vi "move_invader_intensity.vi"(11 "MainCluster_IN":T9) -> (3 "MainCluster_OUT":T9)   [LabVIEW 2019]
uses:
  InitCluster.ctl
  CharacterCluster.ctl
  <vilib>/picture/picture.llb/imagedata.ctl
  ShotInitCluster.ctl
  <vilib>/Utility/miscctls.llb/LVPositionTypeDef.ctl
  <vilib>/Utility/miscctls.llb/LVBoundsTypeDef.ctl
  InvaderPositionArray.ctl
  move_dir_lr.ctl
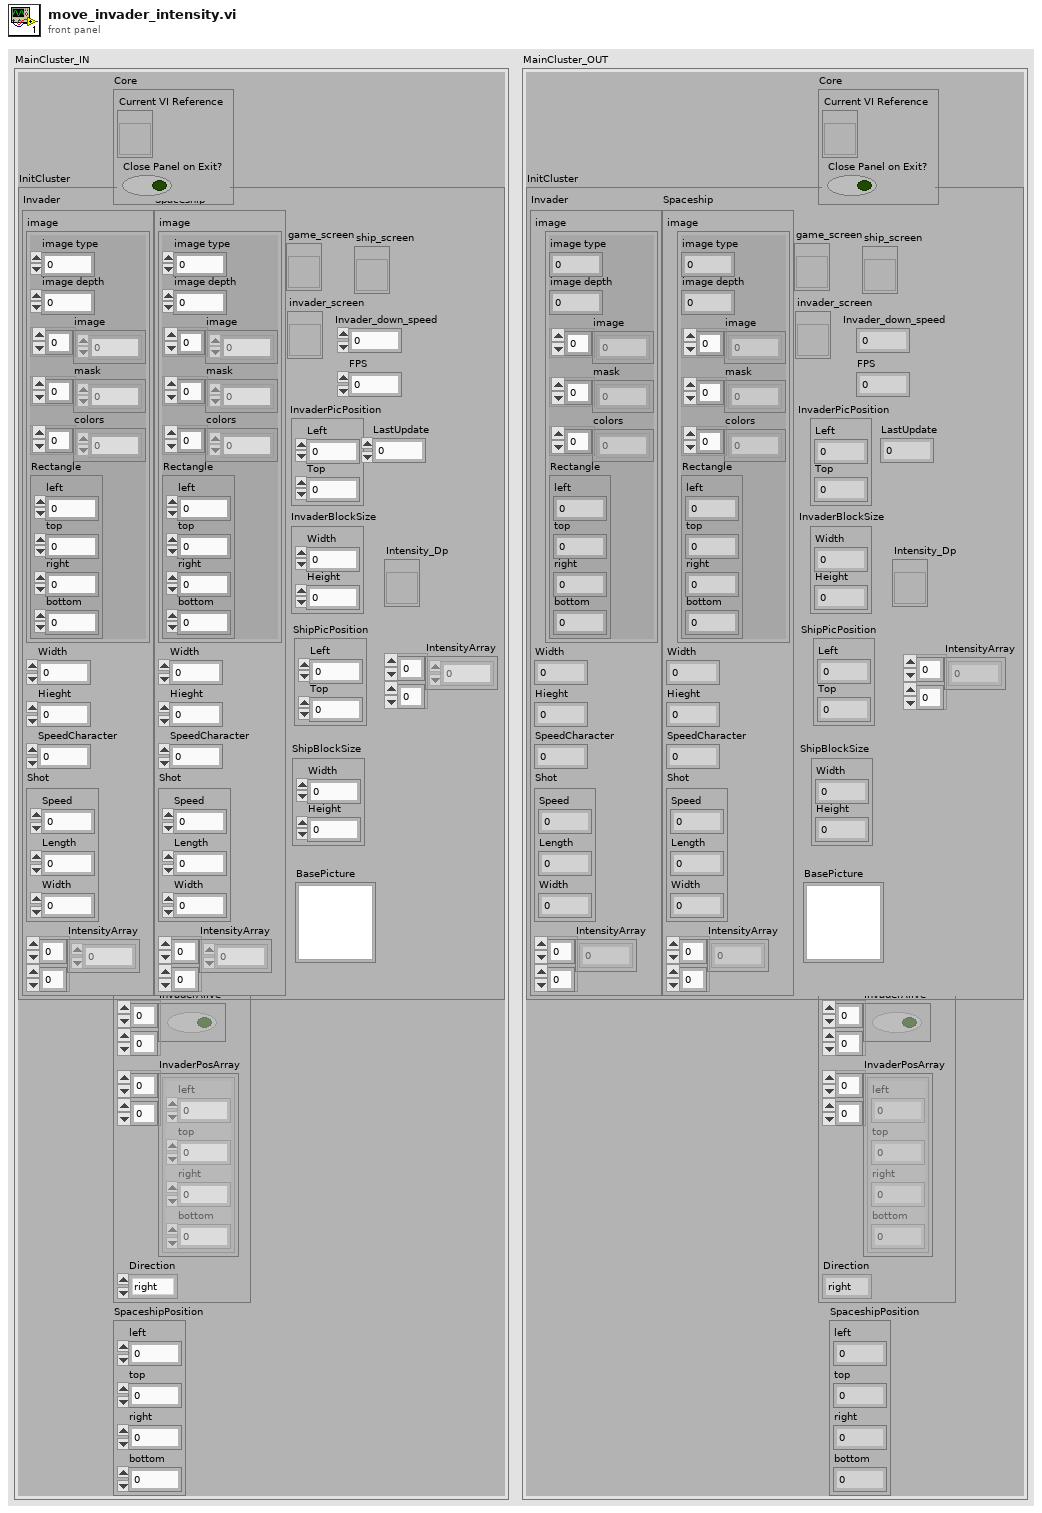
[diagram p1: front panel]
types:
  T1 = typedef "InitCluster.ctl" = cluster{"Invader":T2, "Spaceship":T2, "game_screen":refnum<vi>, "BasePicture":picture, "invader_screen":refnum<vi>, "InvaderPicPosition":T5, "Invader_down_speed":i16, "FPS":u16, "InvaderBlockSize":T6, "ship_screen":refnum<vi>, "ShipBlockSize":T6, "ShipPicPosition":T5, "LastUpdate":u32, "Intensity_Dp":refnum<vi>, "IntensityArray":u8[][]}
  T2 = typedef "CharacterCluster.ctl" = cluster{"image":T3, "Width":u32, "Hieght":u32, "SpeedCharacter":u32, "Shot":T4, "IntensityArray":u8[][]}
  T3 = typedef "imagedata.ctl" = cluster{"image type":i32, "image depth":i32, "image":u8[], "mask":u8[], "colors":u32[], "Rectangle":cluster{"left":i16, "top":i16, "right":i16, "bottom":i16}}
  T4 = typedef "ShotInitCluster.ctl" = cluster{"Speed":u32, "Length":u32, "Width":u32}
  T5 = typedef "LVPositionTypeDef.ctl" = cluster{"Left":i32, "Top":i32}
  T6 = typedef "LVBoundsTypeDef.ctl" = cluster{"Width":u32, "Height":u32}
  T7 = typedef "InvaderPositionArray.ctl" = cluster{"InvaderAlive":bool[][], "InvaderPosArray":cluster{"left":i16, "top":i16, "right":i16, "bottom":i16}[][], "Direction":T8}
  T8 = typedef "move_dir_lr.ctl" = enum16{"right", "left"}
  T9 = cluster{"Core":cluster{"Current VI Reference":refnum<vi>, "Close Panel on Exit?":bool}, "InitCluster":T1, "InvaderPosArray":T7, "SpaceshipPosition":cluster{"left":i16, "top":i16, "right":i16, "bottom":i16}}
  T10 = cluster{"left":i16, "top":i16, "right":i16, "bottom":i16}[][]
  T11 = cluster{"left":i16, "top":i16, "right":i16, "bottom":i16}
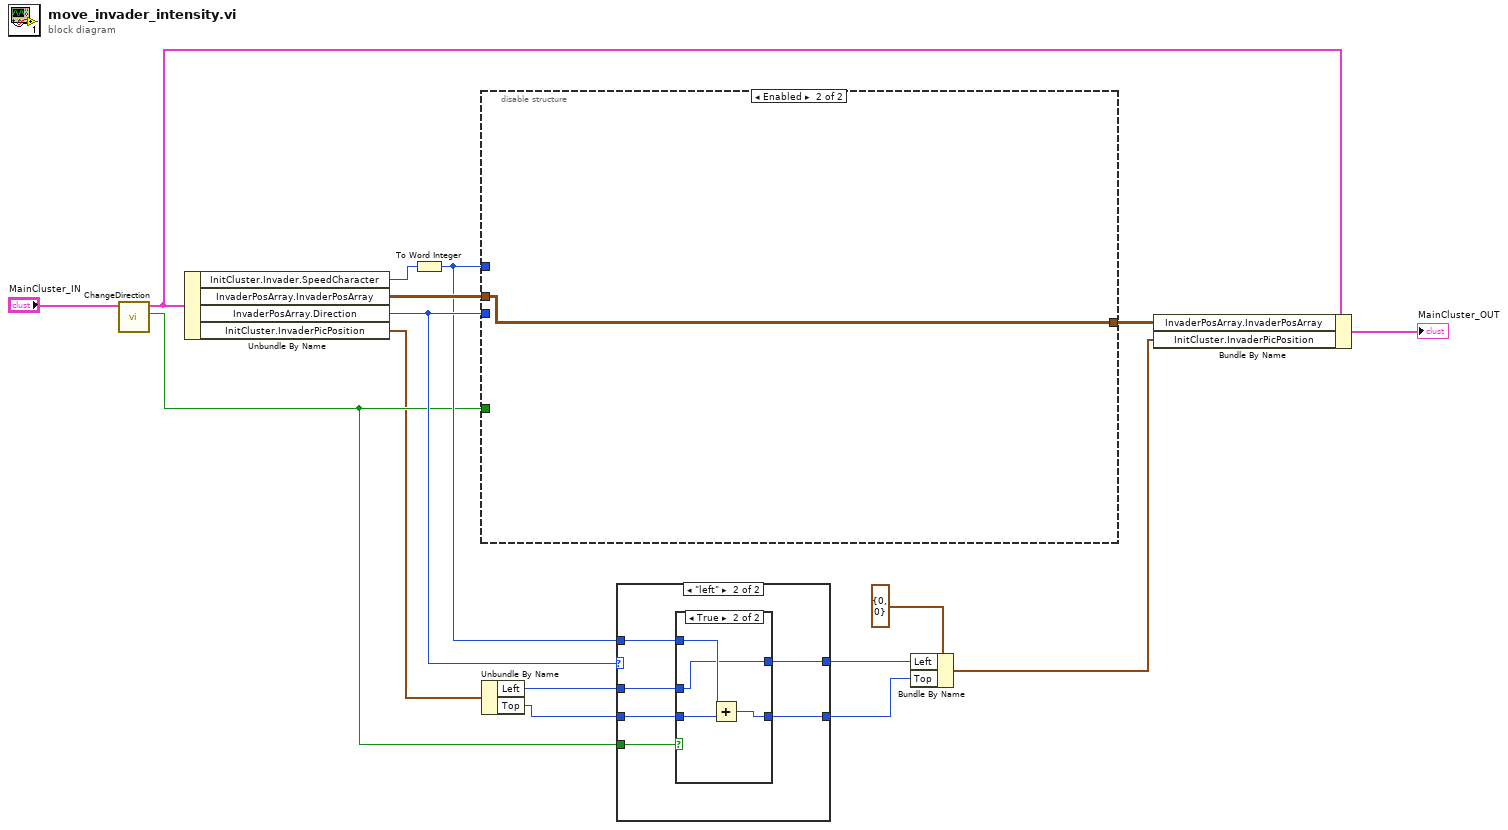
[diagram p0: block diagram]
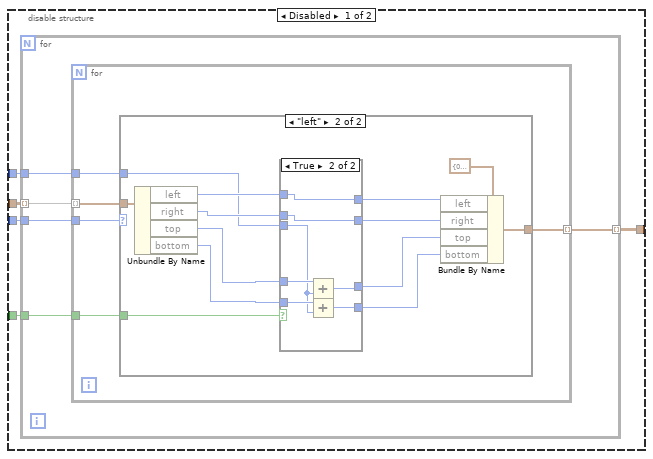
[diagram p2: hidden frame]
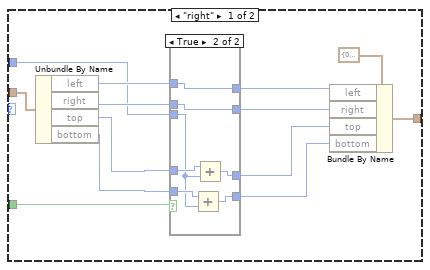
[diagram p3: hidden frame]
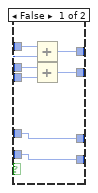
[diagram p4: hidden frame]
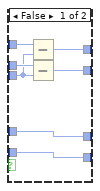
[diagram p5: hidden frame]
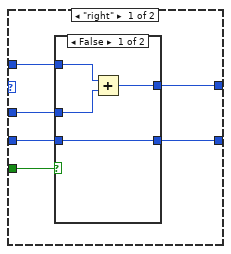
[diagram p6: hidden frame]
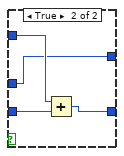
[diagram p7: hidden frame]
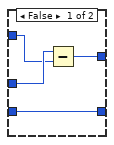
[diagram p8: hidden frame]
diagram:
  n1 = call "ChangeDirection.vi"("MainCluster_IN"="MainCluster_IN") -> ("DirectionChanged"=w8:bool, "MainCluster_OUT"=w13:T9)  [unwired: 9 in]
  n2 = Unbundle By Name(w13) -> ("InitCluster.Invader.SpeedCharacter"=w14:u32, "InvaderPosArray.InvaderPosArray"=w16:T10, "InvaderPosArray.Direction"=w10:T8, "InitCluster.InvaderPicPosition"=w7:T5)
  n3 = To Word Integer(number=w14) -> (16bit integer=w9:i16)
  n4 = disable-structure shown="Enabled" {
    disable-tunnel: w16 -> [w21 w86]
    disable-tunnel: [w20 w86] -> w11
    disable-tunnel: w10 -> [w19 _]
    disable-tunnel: w9 -> [w18 _]
    disable-tunnel: w8 -> [w17 _]
    frame Disabled {
      n5 = for {
        tunnel: w21 -> [w25] mode=indexing
        tunnel: w19 -> [w26]
        tunnel: w17 -> [w24]
        tunnel: w18 -> [w23]
        tunnel: [w22] -> w20 mode=indexing
        n6 = for {
          tunnel: w26 -> [w31]
          tunnel: w25 -> [w30] mode=indexing
          tunnel: w24 -> [w29]
          tunnel: w23 -> [w28]
          tunnel: [w27] -> w22 mode=indexing
          n7 = case shown="\"left\"" w31 {
            tunnel: w30 -> [w44 w71]
            tunnel: [w38 w65] -> w27
            tunnel: w29 -> [w32 w59]
            tunnel: w28 -> [w35 w62]
            frame "right" {
              n8 = Unbundle By Name(w44) -> ("left"=w42:i16, "right"=w40:i16, "top"=w37:i16, "bottom"=w36:i16)
              n9 = case shown="True" w32 {
                tunnel: w42 -> [w51 w58]
                tunnel: [w50 w58] -> w41
                tunnel: w40 -> [w49 w57]
                tunnel: [w48 w57] -> w39
                tunnel: w37 -> [w46 w56]
                tunnel: w36 -> [w45 w55]
                tunnel: w35 -> [w47 w54]
                tunnel: [w46 w53] -> w34
                tunnel: [w45 w52] -> w33
                frame False {
                  n10 = Add(x=w51, y=w47) -> (x+y=w50:i16)
                  n11 = Add(x=w49, y=w47) -> (x+y=w48:i16)
                }
                frame True {
                  n12 = Add(x=w55, y=w54) -> (x+y=w52:i16)
                  n13 = Add(x=w56, y=w54) -> (x+y=w53:i16)
                }
              }
              n14 = Bundle By Name(cluster=T11 {"left"=0, "top"=0, "right"=0, "bottom"=0} ("Rectangle"), "left"=w41, "right"=w39, "top"=w34, "bottom"=w33) -> (w38:T11)
            }
            frame "left" {
              n15 = Unbundle By Name(w71) -> ("left"=w69:i16, "right"=w67:i16, "top"=w64:i16, "bottom"=w63:i16)
              n16 = case shown="True" w59 {
                tunnel: w69 -> [w78 w85]
                tunnel: [w77 w85] -> w68
                tunnel: w67 -> [w76 w84]
                tunnel: [w75 w84] -> w66
                tunnel: w64 -> [w73 w82]
                tunnel: w63 -> [w72 w81]
                tunnel: w62 -> [w74 w79]
                tunnel: [w73 w83] -> w61
                tunnel: [w72 w80] -> w60
                frame False {
                  n17 = Subtract(x=w78, y=w74) -> (x-y=w77:i16)
                  n18 = Subtract(x=w76, y=w74) -> (x-y=w75:i16)
                }
                frame True {
                  n19 = Add(x=w82, y=w79) -> (x+y=w83:i16)
                  n20 = Add(x=w81, y=w79) -> (x+y=w80:i16)
                }
              }
              n21 = Bundle By Name(cluster=T11 {"left"=0, "top"=0, "right"=0, "bottom"=0} ("Rectangle"), "left"=w68, "right"=w66, "top"=w61, "bottom"=w60) -> (w65:T11)
            }
          }
        }
      }
    }
    frame Enabled {
    }
  }
  n22 = Unbundle By Name(w7) -> ("Left"=w6:i32, "Top"=w5:i32)
  n23 = case shown="\"left\"" w10 {
    tunnel: w6 -> [w91 w106]
    tunnel: w9 -> [w92 w105]
    tunnel: [w90 w104] -> w3
    tunnel: w8 -> [w89 w103]
    tunnel: w5 -> [w88 w102]
    tunnel: [w87 w101] -> w2
    frame "right" {
      n24 = case shown="False" w89 {
        tunnel: w92 -> [w96 w100]
        tunnel: w91 -> [w95 w98]
        tunnel: [w94 w98] -> w90
        tunnel: w88 -> [w93 w99]
        tunnel: [w93 w97] -> w87
        frame False {
          n25 = Add(x=w96, y=w95) -> (x+y=w94:i32)
        }
        frame True {
          n26 = Add(x=w100, y=w99) -> (x+y=w97:i32)
        }
      }
    }
    frame "left" {
      n27 = case shown="True" w103 {
        tunnel: w106 -> [w110 w111]
        tunnel: w105 -> [w109 w114]
        tunnel: [w108 w111] -> w104
        tunnel: w102 -> [w107 w113]
        tunnel: [w107 w112] -> w101
        frame False {
          n28 = Subtract(x=w110, y=w109) -> (x-y=w108:i32)
        }
        frame True {
          n29 = Add(x=w114, y=w113) -> (x+y=w112:i32)
        }
      }
    }
  }
  n30 = Bundle By Name(cluster=T5 {"Left"=0, "Top"=0} ("InitCluster.InvaderPicPosition"), "Left"=w3, "Top"=w2) -> (w1:T5)
  n31 = Bundle By Name(cluster=w13, "InvaderPosArray.InvaderPosArray"=w11, "InitCluster.InvaderPicPosition"=w1) -> (→"MainCluster_OUT":T9)
